vi "Parse Gcode.vi"(8 "error in (no error)":errorcluster, 10 "Read Coordinates":path, 11 "Stage Actor.lvlib:Stage.lvclass":refnum<class "Stage.lvclass">) -> (0 "error out":errorcluster, 3 "Stage Actor.lvlib:Stage.lvclass":refnum<class "Stage.lvclass">)   [LabVIEW 2018, in "Stage Actor.lvlib" / "Stage.lvclass"]
uses:
  Stage.lvclass
  Stage.lvclass/Stage.ctl
  <vilib>/Utility/file.llb/Read Delimited Spreadsheet (string).vi
  Stage Actor.lvlib
panel:
  out "Line Data":T1
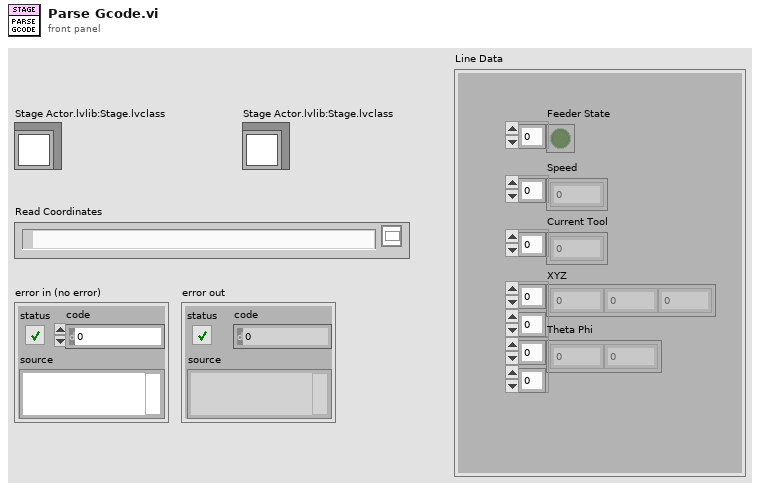
[diagram p1: front panel]
types:
  T1 = cluster{"XYZ":dbl[][], "Theta Phi":dbl[][], "Current Tool":i16[], "Speed":dbl[], "Feeder State":bool[]}
  T2 = cluster{"Print Data":cluster{"XYZ":dbl[][], "Theta Phi":dbl[][], "Current Tool":i16[], "Speed":dbl[], "Feeder State":bool[]}, "Task":string}
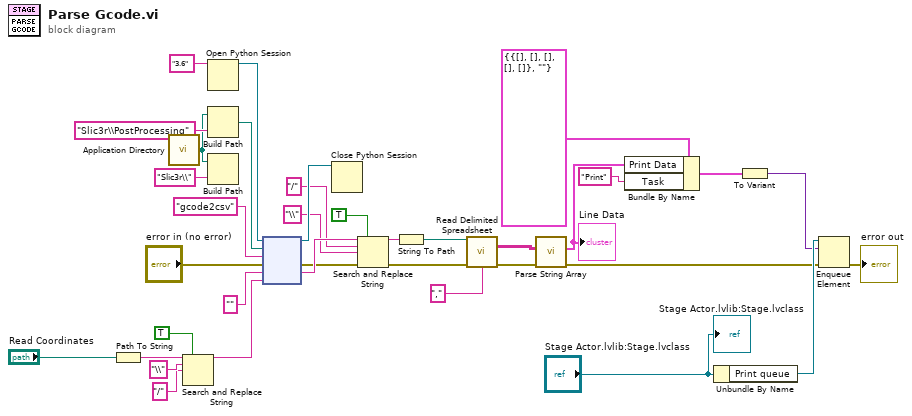
[diagram p0: block diagram]
diagram:
  n1 = Path To String(path="Read Coordinates") -> (string=w26:string)
  n2 = call <vilib>:"Application Directory.vi"() -> ("Application Directory"=w29:path)
  n3 = Search and Replace String(replace all?=TRUE ("replace all? (F)"), input string=w26, search string="\\", replace string="/" ("replace string (\"\")")) -> (result string=w23:string)  [unwired: 4 in, 3 out]
  n4 = Open Python Session(python version="3.6" ("Python version")) -> (session out=w36:refnum<k35>)  [unwired: 2 in, 1 out]
  n5 = Build Path(base path=w29, name or relative path="Slic3r\\PostProcessing") -> (appended path=w33:path)
  n6 = Build Path(base path=w29, name or relative path="Slic3r\\") -> ()  [unwired: 1 out]
  n7 = node(w36, w33, "gcode2csv" ("function name"), "error in (no error)", "", w23) -> (w34:refnum<k35>, w5:errorcluster, w21:string)  [unwired: 1 in, 2 out]
  n8 = Close Python Session(session in=w34) -> ()  [unwired: 1 in, 1 out]
  n9 = Search and Replace String(replace all?=TRUE ("replace all? (F)"), input string=w21, search string="/", replace string="\\" ("replace string (\"\")"), error in=w5) -> (result string=w20:string, error out=w4:errorcluster)  [unwired: 3 in, 2 out]
  n10 = String To Path(string=w20) -> (path=w16:path)
  n11 = call-poly <vilib>:"Read Delimited Spreadsheet.vi"("file path (dialog if empty)"=w16, "error in (no error)"=w4, "delimiter (\\t)"="," ("delimiter (\\t)")) -> ("all rows"=w15:string[][], "error out"=w3:errorcluster)  [unwired: 7 in, 4 out]
  n12 = call "Parse String Array.vi"("error in (no error)"=w3, "String XYZ"=w15) -> ("error out"=w2:errorcluster, "Line Data"=w11:T1)  [unwired: 8 in]
  "Line Data" <- w11
  n13 = Bundle By Name(cluster=T2 {"Print Data"={"XYZ"=[], "Theta Phi"=[], "Current Tool"=[], "Speed"=[], "Feeder State"=[]}, "Task"=""} ("Print Message"), "Print Data"=w11, "Task"="Print") -> (w9:T2)
  n14 = Unbundle By Name("Stage Actor.lvlib:Stage.lvclass") -> ("Print queue"=w13:refnum<queue>)
  n15 = To Variant(anything=w9) -> (Variant=w8:variant)
  n16 = Enqueue Element(queue=w13, element=w8, error in (no error)=w2) -> (error out=→"error out":errorcluster)  [unwired: 1 in, 2 out]
  "Stage Actor.lvlib:Stage.lvclass" <- "Stage Actor.lvlib:Stage.lvclass"
